vi "process safe state.vi"(8 "error in":errorcluster, 9 "result allocation":T1, 10 "parameters":T1, 11 "module in":refnum<class "TEST RUNTIME.lvclass">) -> (0 "error out":errorcluster, 1 "results":T1, 2 "parameter allocation":T1, 3 "module out":refnum<class "TEST RUNTIME.lvclass">)   [LabVIEW 2013, in "configuration tests.lvlib" / "TEST RUNTIME.lvclass"]
doc: "Provides an interface for information processing by a module when in a safe state. This interface simply calls the normal processing function. However, if child modules need to have custom logic during safe-state operation, this can be implemented here.\nNI Tag Bus Module Framework 1.0.2.34\nNI Systems Engineering"
uses:
  TEST RUNTIME.lvclass
  <vilib>/NI/Tag Bus/table/data table.ctl
  TEST RUNTIME.lvclass/TEST RUNTIME.ctl
  <vilib>/NI/Tag Bus/table/data polymorphs/write one/write Double.vi
  <vilib>/NI/Tag Bus/table/data table.lvlib
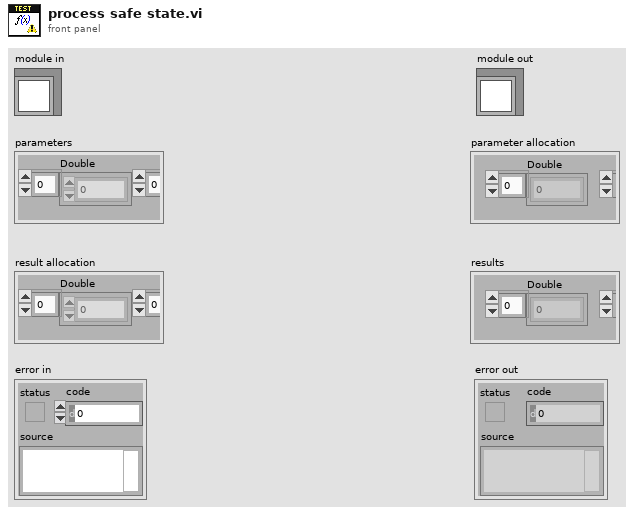
[diagram p1: front panel]
types:
  T1 = typedef "tag bus.lvlib/data table.lvlib/data table.ctl" = cluster{"Double":dbl[], "Single":sgl[], "I64":i64[], "I32":i32[], "I16":i16[], "I8":i8[], "U64":u64[], "U32":u32[], "U16":u16[], "U8":u8[], "Boolean":bool[], "String":string[], "Array of Double":cluster{"DBL Array":dbl[]}[], "Array of Single":cluster{"SGL Array":sgl[]}[], "Array of I64":cluster{"I64 Array":i64[]}[], "Array of I32":cluster{"I32 Array":i32[]}[], "Array of I16":cluster{"I16 Array":i16[]}[], "Array of I8":cluster{"I8 Array":i8[]}[], "Array of U64":cluster{"U64 Array":u64[]}[], "Array of U32":cluster{"U32 Array":u32[]}[], "Array of U16":cluster{"U16 Array":u16[]}[], "Array of U8":cluster{"U8 Array":u8[]}[], "Array of Boolean":cluster{"Boolean Array":bool[]}[], "Array of String":cluster{"String Array":string[]}[]}
  T2 = typedef "configuration tests.lvlib/TEST RUNTIME.lvclass/state control.ctl" = cluster{"state":u8, "control index (dbl)":i32, "output index (dbl)":i32}
  T3 = typedef "configuration tests.lvlib/TEST RUNTIME.lvclass/control module.ctl" = cluster{"setpoint index (dbl)":i32, "proc var index (dbl)":i32, "output index (dbl)":i32, "output range":cluster{"output high":dbl, "output low":dbl}, "Kp":dbl, "Ki":dbl, "Kd":dbl, "error int":dbl, "last error":dbl}
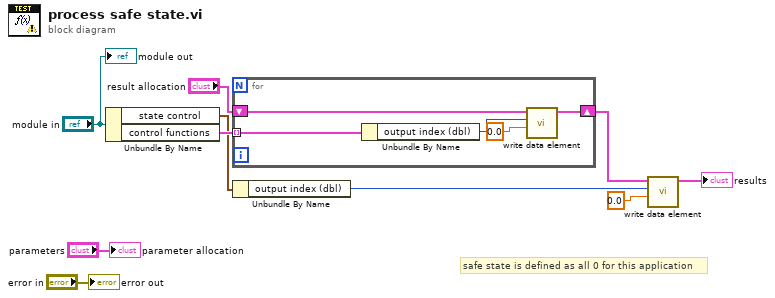
[diagram p0: block diagram]
diagram:
  # "safe state is defined as all 0 for this application"
  n1 = Unbundle By Name("module in") -> ("state control"=w5:T2, "control functions"=w7:T3[])
  n2 = for {
    shift-right: [w12] -> w4
    shift-left: "result allocation" -> [w14]
    tunnel: w7 -> [w15] mode=indexing
    n3 = Unbundle By Name(w15) -> ("output index (dbl)"=w13:i32)
    n4 = call-poly <vilib>:"write data element.vi"("value"=0.0, "index"=w13, "data table in"=w14) -> ("data table out"=w12:T1)  [unwired: 8 in]
  }
  n5 = Unbundle By Name(w5) -> ("output index (dbl)"=w3:i32)
  n6 = call-poly <vilib>:"write data element.vi"("value"=0.0, "index"=w3, "data table in"=w4) -> ("data table out"=→"results":T1)  [unwired: 8 in]
  "module out" <- "module in"
  "error out" <- "error in"
  "parameter allocation" <- "parameters"
